vi "AMZ_S3_APIHLP_Parse Bucket Versioning Configuration.vi"(8 "error in (no error)":errorcluster, 10 "Response body":string) -> (0 "error out":errorcluster, 3 "VersioningConfiguration":T1)   [LabVIEW 2015, in "LV Interface for Amazon S3.lvlib"]
uses:
  LV Interface for Amazon S3.lvlib
  Typedefs/AMZ_S3_API_VersioningConfiguration.ctl
  Typedefs/AMZ_S3_Versioning Status.ctl
  Typedefs/AMZ_S3_MFA Delete.ctl
  XML Parser/XML Parser.lvlib
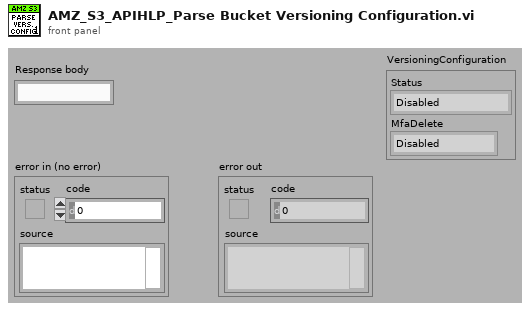
[diagram p1: front panel]
types:
  T1 = typedef "LV Interface for Amazon S3.lvlib/AMZ_S3_API_VersioningConfiguration.ctl" = cluster{"Status":T2, "MfaDelete":T3}
  T2 = typedef "LV Interface for Amazon S3.lvlib/AMZ_S3_Versioning Status.ctl" = enum16{"Disabled", "Suspended", "Enabled"}
  T3 = typedef "LV Interface for Amazon S3.lvlib/AMZ_S3_MFA Delete.ctl" = enum16{"Disabled", "Enabled"}
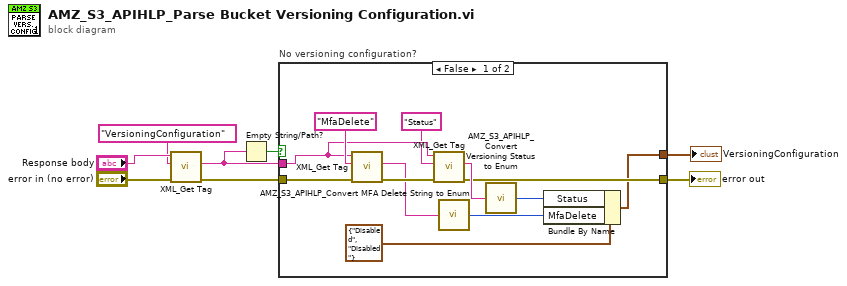
[diagram p0: block diagram]
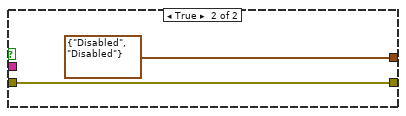
[diagram p2: hidden frame]
diagram:
  n1 = call "XML_Get Tag.vi"("error in (no error)"="error in (no error)", "Tag name"="VersioningConfiguration", "XML String in"="Response body") -> ("error out"=w3:errorcluster, "Tag value"=w4:string)  [unwired: 4 in, 3 out]
  n2 = Empty String/Path?(string/path=w4) -> (empty?=w5:bool)
  n3 = case "No versioning configuration?" shown="False" w5 {
    tunnel: w4 -> [w17 _]
    tunnel: w3 -> [w20 w22]
    tunnel: [w10 w22] -> w2
    tunnel: [w9 T1 {"Status"=enum."Disabled", "MfaDelete"=enum."Disabled"} ("VersioningConfiguration")] -> w1
    frame False {
      n4 = call "XML_Get Tag.vi"("error in (no error)"=w20, "Tag name"="MfaDelete", "XML String in"=w17) -> ("error out"=w18:errorcluster, "Tag value"=w14:string)  [unwired: 4 in, 3 out]
      n5 = call "XML_Get Tag.vi"("error in (no error)"=w18, "Tag name"="Status", "XML String in"=w17) -> ("error out"=w10:errorcluster, "Tag value"=w12:string)  [unwired: 4 in, 3 out]
      n6 = call "AMZ_S3_APIHLP_Convert MFA Delete String to Enum.vi"("MFA Delete String"=w14) -> ("MFA Delete"=w13:T3)  [unwired: 4 in]
      n7 = call "AMZ_S3_APIHLP_Convert Versioning Status to Enum.vi"("Status String"=w12) -> ("Status"=w11:T2)  [unwired: 4 in]
      n8 = Bundle By Name(cluster=T1 {"Status"=enum."Disabled", "MfaDelete"=enum."Disabled"} ("VersioningConfiguration"), "Status"=w11, "MfaDelete"=w13) -> (w9:T1)
    }
    frame True {
    }
  }
  "error out" <- w2
  "VersioningConfiguration" <- w1
